vi "Stop Core.vi"(10 "final error code":i32, 11 "LED Matrix in":refnum<class "LED Matrix.lvclass">) -> (3 "LED Matrix out":refnum<class "LED Matrix.lvclass">)   [LabVIEW 2026, in "LED Matrix.lvlib" / "LED Matrix.lvclass"]
doc: "<p>(<strong>Filename</strong>: <span class=\"dnl\">Actor Framework.lvlib:Actor.lvclass:Stop Core.vi</span>)</p>\n<p>Defines what the actor does before it stops. Use the <strong>final error code</strong> input to determine whether the actor shut down in response to an error.</p>\n<p>By default, this method passes the Stop message along to all <a href=\"nihelplauncher://docs/csh?context=lvcore_lvcomm_af_launch_nested_actor\">auto-stop nested actors</a>. A descendant class may override this method to define additional behavior, such as shutting down any processes the actor initiated in its override of the <a href=\"nihelplauncher://docs/csh?context=lvcore_lvcomm_af_actor_core\">Actor Core</a> method.</p>"
uses:
  LED Matrix.lvclass
  LED Matrix.lvclass/LED Matrix.ctl
  <vilib>/ActorFramework/Actor/Actor.lvclass
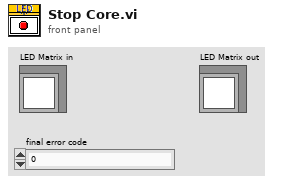
[diagram p1: front panel]
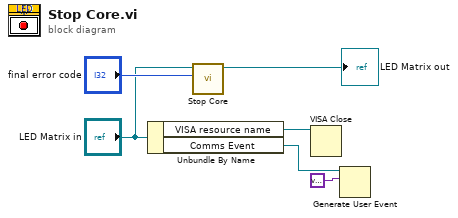
[diagram p0: block diagram]
diagram:
  n1 = Unbundle By Name("LED Matrix in") -> ("VISA resource name"=w1:refnum<visa-resource-name>, "Comms Event"=w2:refnum<user-event>)
  n2 = call-parent "Stop Core.vi"("final error code"="final error code", "Actor in"="LED Matrix in") -> ("Actor out"=→"LED Matrix out":refnum<class "LED Matrix.lvclass">)  [unwired: 9 in]
  n3 = VISA Close(VISA resource name=w1) -> ()  [unwired: 1 in, 1 out]
  n4 = Generate User Event(user event=w2, event data cluster=variant ("event data")) -> ()  [unwired: 2 in, 2 out]
